vi "KN-OptionsToString -矩形.vi"(0 "Rectangle 3":T5 {"Rotation" format="%.2f"; "Left" scale=0.0..1024.0; "Right" scale=0.0..1024.0}, 1 "Options IN":T3={"Search Direction"=2, "Edge Options"={"Edge Polarity"=0, "Kernel Size"=3, "Width"=3, "Minimum Edge Strength"=50.0, "Interpolation Type"=enum."Bilinear Fixed", "Data Processing Method"=enum."Average"}} {"Search Direction" items=["Left to Right", "Right to Left", "Top to Bottom", "Bottom to Top"]; "Edge Options"."Edge Polarity" items=["All Edges", "Rising Edges", "Falling Edges"]; "Edge Options"."Minimum Edge Strength" format="%.2f"; "Edge Options"."Width" step=2; "Edge Options"."Kernel Size" step=2}, 3 "(Color Threshold 1)":cluster{"Lower value":i32, "Upper value":i32}={"Lower value"=12, "Upper value"=253}) -> (14 "OptionsString Out":string=";1480.000;1115.000;378.000;757.000;0.000;0.000;0;1;3;3;10.000;4;0;1;1;1;1;65280;255;16776960;16711680;;3;10;3;23;255")   [LabVIEW 2015]
uses:
  <vilib>/vision/Measure.llb/Edge Options.ctl
  <vilib>/vision/Measure.llb/Edge Polarity.ctl
panel:
  out "Contours":T4(array[cluster])
  out "Array":string[](array[string])
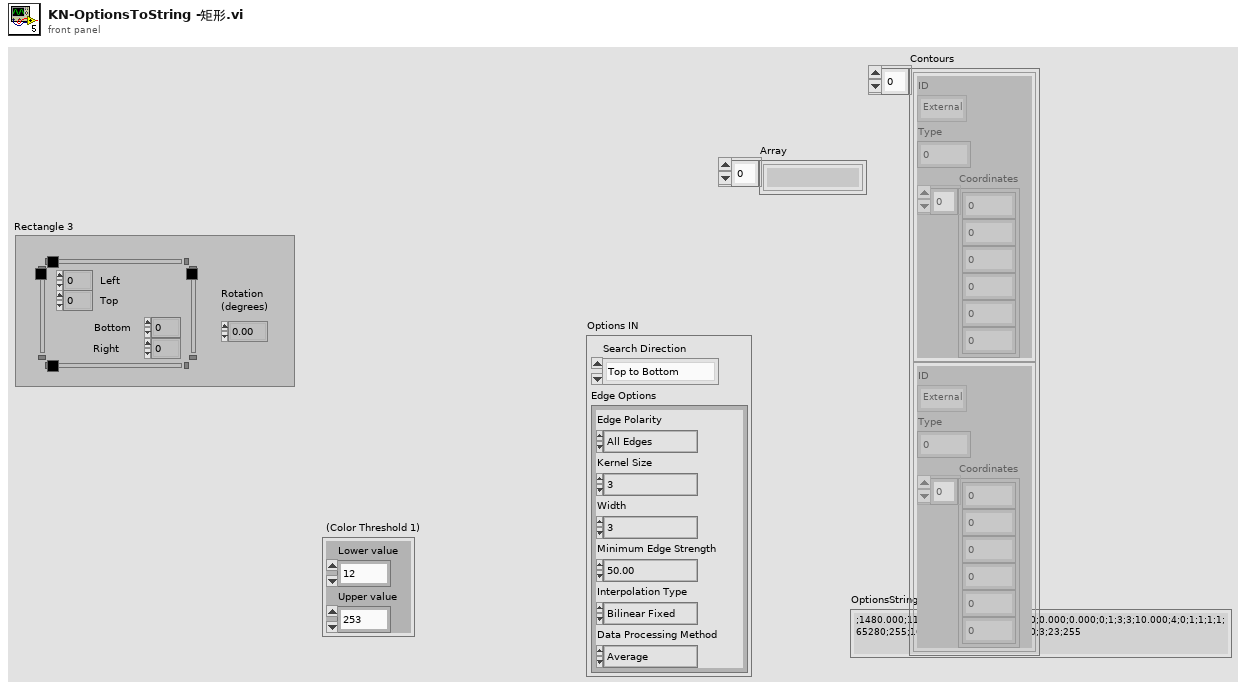
[diagram p1: front panel]
types:
  T1 = typedef "Edge Options.ctl" = cluster{"Edge Polarity":T2, "Kernel Size":u32, "Width":u32, "Minimum Edge Strength":sgl, "Interpolation Type":enum32{"Zero Order", "Bilinear", "Quadratic", "Cubic", "Bilinear Fixed"}, "Data Processing Method":enum32{"Average", "Median"}}
  T2 = typedef "Edge Polarity.ctl" = u32
  T3 = cluster{"Search Direction":u32, "Edge Options":T1}
  T4 = cluster{"ID":enum32{"External", "Internal"}, "Type":u32, "Coordinates":i32[]}[]
  T5 = typedef "IMAQ Rectangle" = cluster{"Left":i32, "Top":i32, "Right":i32, "Bottom":i32, "Rotation":dbl}
  T6 = cluster{"Edge Options":T1, "Show Search Area":bool, "Show Search Lines":bool, "Show Edges Found":bool, "Show Result":bool, "Search Area Color":u32, "Search Lines Color":u32, "Edge Locations Color":u32, "Result Color":u32, "Overlay Group Name":string, "Search Direction":u32}
  T7 = typedef "ROI Descriptor" = cluster{"Global Rectangle":i32[], "Contours":cluster{"ID":enum32{"External", "Internal"}, "Type":u32, "Coordinates":i32[]}[]}
  T8 = cluster{"Lower value":string, "Upper value":string}
  T9 = cluster{"ID":enum32{"External", "Internal"}, "Type":u32, "Coordinates":i32[]}
  T10 = enum32{"Zero Order", "Bilinear", "Quadratic", "Cubic", "Bilinear Fixed"}
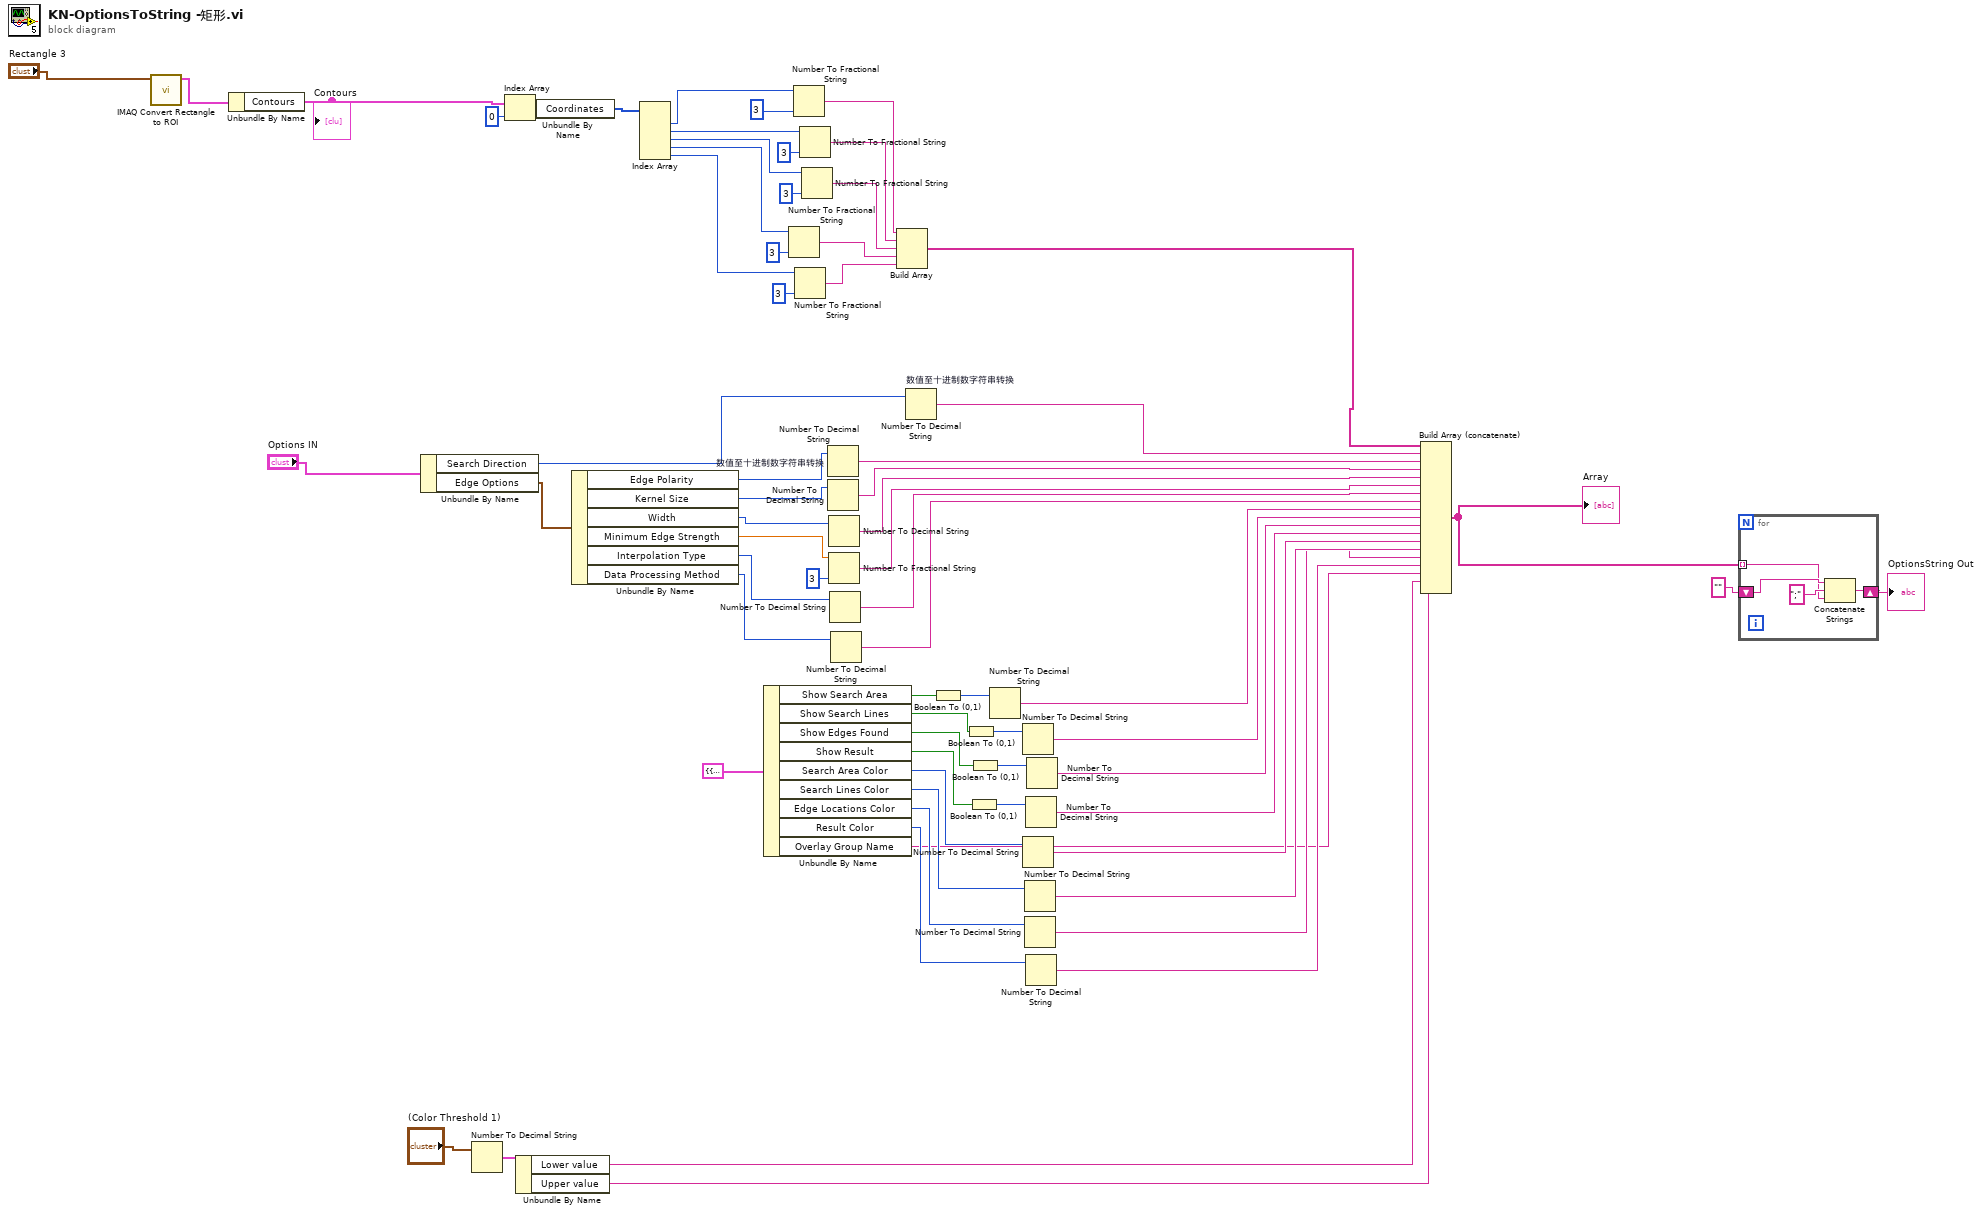
[diagram p0: block diagram]
diagram:
  n1 = call "IMAQ Convert Rectangle to ROI"("Rectangle"="Rectangle 3") -> ("ROI Descriptor"=w2:T7)  [unwired: 8 in, 1 out]
  n2 = Unbundle By Name(w2) -> ("Contours"=w23:T4)
  "Contours" <- w23
  n3 = Unbundle By Name("Options IN") -> ("Search Direction"=w29:u32, "Edge Options"=w43:T1)
  n4 = Number To Decimal String(number="(Color Threshold 1)") -> (decimal integer string=w26:T8)  [unwired: 1 in]
  n5 = Index Array(array=w23, index=0 ("索引")) -> (element=w21:T9)
  n6 = Unbundle By Name(w26) -> ("Lower value"=w25:string, "Upper value"=w24:string)
  n7 = Unbundle By Name(w21) -> ("Coordinates"=w20:i32[])
  n8 = Unbundle By Name(w43) -> ("Edge Polarity"=w41:T2, "Kernel Size"=w40:u32, "Width"=w39:u32, "Minimum Edge Strength"=w38:sgl, "Interpolation Type"=w37:T10, "Data Processing Method"=w36:enum32{"Average", "Median"})
  n9 = Index Array(array=w20) -> (element #1=w19:i32, element #2=w13:i32, element #3=w12:i32, element #4=w11:i32, element #5=w10:i32)  [unwired: 5 in]
  n10 = Unbundle By Name(T6 {"Edge Options"={"Edge Polarity"=0, "Kernel Size"=0, "Width"=0, "Minimum Edge Strength"=0.0, "Interpolation Type"=enum."Bilinear Fixed", "Data Processing Method"=enum."Average"}, "Show Search Area"=TRUE, "Show Search Lines"=FALSE, "Show Edges Found"=FALSE, "Show Result"=TRUE, "Search Area Color"=65280, "Search Lines Color"=255, "Edge Locations Color"=16776960, "Result Color"=16711680, "Overlay Group Name"="", "Search Direction"=2} ("Options (Find Circular Edge 1)")) -> ("Show Search Area"=w67:bool, "Show Search Lines"=w62:bool, "Show Edges Found"=w61:bool, "Show Result"=w60:bool, "Search Area Color"=w59:u32, "Search Lines Color"=w58:u32, "Edge Locations Color"=w57:u32, "Result Color"=w56:u32, "Overlay Group Name"=w47:string)
  n11 = Number To Fractional String(number=w11, precision (6)=i16 3 ("精度(6)")) -> (F-format string=w6:string)  [unwired: 2 in]
  n12 = Number To Fractional String(number=w19, precision (6)=i16 3 ("精度(6)")) -> (F-format string=w9:string)  [unwired: 2 in]
  n13 = Number To Fractional String(number=w10, precision (6)=i16 3 ("精度(6)")) -> (F-format string=w5:string)  [unwired: 2 in]
  n14 = Number To Fractional String(number=w13, precision (6)=i16 3 ("精度(6)")) -> (F-format string=w8:string)  [unwired: 2 in]
  n15 = Number To Fractional String(number=w12, precision (6)=i16 3 ("精度(6)")) -> (F-format string=w7:string)  [unwired: 2 in]
  n16 = Number To Decimal String "数值至十进制数字符串转换"(number=w41) -> (decimal integer string=w35:string)  [unwired: 1 in]
  n17 = Number To Decimal String(number=w40) -> (decimal integer string=w34:string)  [unwired: 1 in]
  n18 = Number To Decimal String(number=w39) -> (decimal integer string=w33:string)  [unwired: 1 in]
  n19 = Number To Fractional String(number=w38, precision (6)=i16 3 ("精度(6)")) -> (F-format string=w32:string)  [unwired: 2 in]
  n20 = Number To Decimal String(number=w37) -> (decimal integer string=w31:string)  [unwired: 1 in]
  n21 = Number To Decimal String(number=w36) -> (decimal integer string=w30:string)  [unwired: 1 in]
  n22 = Build Array(w9, w8, w7, w6, w5) -> (w4:string[])
  n23 = Number To Decimal String "数值至十进制数字符串转换"(number=w29) -> (decimal integer string=w28:string)  [unwired: 1 in]
  n24 = Boolean To (0,1)(Boolean=w67) -> (0, 1=w66:i16)
  n25 = Boolean To (0,1)(Boolean=w62) -> (0, 1=w65:i16)
  n26 = Boolean To (0,1)(Boolean=w60) -> (0, 1=w63:i16)
  n27 = Boolean To (0,1)(Boolean=w61) -> (0, 1=w64:i16)
  n28 = Number To Decimal String(number=w66) -> (decimal integer string=w55:string)  [unwired: 1 in]
  n29 = Number To Decimal String(number=w65) -> (decimal integer string=w54:string)  [unwired: 1 in]
  n30 = Number To Decimal String(number=w59) -> (decimal integer string=w51:string)  [unwired: 1 in]
  n31 = Number To Decimal String(number=w58) -> (decimal integer string=w50:string)  [unwired: 1 in]
  n32 = Number To Decimal String(number=w57) -> (decimal integer string=w49:string)  [unwired: 1 in]
  n33 = Number To Decimal String(number=w63) -> (decimal integer string=w52:string)  [unwired: 1 in]
  n34 = Number To Decimal String(number=w56) -> (decimal integer string=w48:string)  [unwired: 1 in]
  n35 = Number To Decimal String(number=w64) -> (decimal integer string=w53:string)  [unwired: 1 in]
  n36 = Build Array (concatenate)(w4, w28, w35, w34, w33, w32, w31, w30, w55, w54, w53, w52, w51, w50, w49, w48, w47, w25, w24) -> (w45:string[])
  "Array" <- w45
  n37 = for {
    tunnel: w45 -> [w69] mode=indexing
    shift-right: [w72] -> w44
    shift-left: "" -> [w70]
    n38 = Concatenate Strings(w70, ";" ("字符串"), w69) -> (w72:string)
  }
  "OptionsString Out" <- w44
